vi "svc_Check for Waveform Parameter Continuity (no state).vi"(0 "scaled signal [EU]":waveform(dbl), 2 "checks for channel parameter change":T4, 5 "error in (no error)":errorcluster, 6 "reset":bool, 7 "expected channel info":T1={"sensor sensitivity"=1000.0, "engineering units"=1, "dB reference"=1.0, "custom label"="EU", "weighting filter"=0, "pregain"=0.0} {"pregain" format="%.2f"; "weighting filter" items=["Linear", "A-weighting", "B-weighting", "C-weighting", "ITU-R 468-4", "Dolby", "CCITT", "C-message", "Wb", "Wc", "Wd", "We", "Wf", "Wh", "Wj", "Wk", "Wm", "AES17 20 kHz lowpass", "AES17 40 kHz lowpass", "AES17 20 kHz highpass", "AES17 40 kHz highpass"]; "dB reference" format="%^.1e"; "engineering units" items=["custom..."=0, "V"=1, "A"=21, "C"=30, "pC"=31, "s"=32, "-"=29, "Pa"=2, "N"=20, "g"=3, "m/s^2"=4, "m/s"=5, "m"=6, "mm/s"=12, "mm"=13, "micron/s"=14, "micron"=15, "in/s^2"=7, "in/s"=8, "in"=9, "mil/s"=10, "mil"=11, "rad/s^2"=16, "rad/s"=17, "rad"=18, "deg/s^2"=26, "deg/s"=27, "deg"=28, "RPM"=22, "cycle/s^2"=23, "Hz"=24, "cycle"=25, "strain"=19]; "sensor sensitivity" format="%#_5f"}, 8 "channel index":i32, 9 "expected waveform parameters":T5) -> (11 "next expected waveform parameters":T5, 13 "next expected channel info":T1={"sensor sensitivity"=1000.0, "engineering units"=1, "dB reference"=1.0, "custom label"="EU", "weighting filter"=0, "pregain"=0.0} {"pregain" format="%.2f"; "weighting filter" items=["Linear", "A-weighting", "B-weighting", "C-weighting", "ITU-R 468-4", "Dolby", "CCITT", "C-message", "Wb", "Wc", "Wd", "We", "Wf", "Wh", "Wj", "Wk", "Wm", "AES17 20 kHz lowpass", "AES17 40 kHz lowpass", "AES17 20 kHz highpass", "AES17 40 kHz highpass"]; "dB reference" format="%^.1e"; "engineering units" items=["custom..."=0, "V"=1, "A"=21, "C"=30, "pC"=31, "s"=32, "-"=29, "Pa"=2, "N"=20, "g"=3, "m/s^2"=4, "m/s"=5, "m"=6, "mm/s"=12, "mm"=13, "micron/s"=14, "micron"=15, "in/s^2"=7, "in/s"=8, "in"=9, "mil/s"=10, "mil"=11, "rad/s^2"=16, "rad/s"=17, "rad"=18, "deg/s^2"=26, "deg/s"=27, "deg"=28, "RPM"=22, "cycle/s^2"=23, "Hz"=24, "cycle"=25, "strain"=19]; "sensor sensitivity" format="%#_5f"}, 14 "dup scaled signal [EU]":waveform(dbl), 15 "waveform parameter changed":bool, 16 "dt":dbl, 17 "array length":i32, 19 "error out":errorcluster)   [LabVIEW 2017]
uses:
  <vilib>/addons/_NISVFA/_Shared subVIs/Controls/svc_Waveform Parameters.ctl
  <vilib>/addons/_NISVFA/_Shared subVIs/Controls/svc_Channel Info.ctl
  <vilib>/addons/_NISVFA/_Shared subVIs/Controls/svc_Engineering Units Text Ring.ctl
  <vilib>/addons/_NISVFA/_Shared subVIs/Controls/svc_Weighting Filter Text Ring.ctl
  <vilib>/addons/_NISVFA/_Shared subVIs/Common/svc_Engineering Units to Unit Label.vi
  <vilib>/addons/_NISVFA/_Shared subVIs/Common/svc_Unit Label to Engineering Units.vi
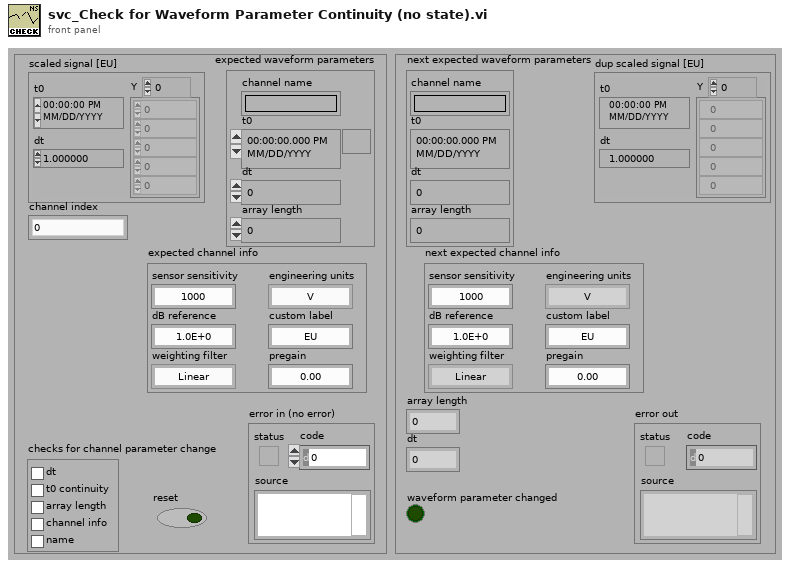
[diagram p1: front panel]
types:
  T1 = typedef "svc_Channel Info.ctl" = cluster{"sensor sensitivity":dbl, "engineering units":T2, "dB reference":dbl, "custom label":string, "weighting filter":T3, "pregain":dbl}
  T2 = typedef "svc_Engineering Units Text Ring.ctl" = u16
  T3 = typedef "svc_Weighting Filter Text Ring.ctl" = u16
  T4 = cluster{"dt":bool, "t0 continuity":bool, "array length":bool, "channel info":bool, "name":bool}
  T5 = typedef "svc_Waveform Parameters.ctl" = cluster{"channel name":string, "t0":timestamp, "dt":dbl, "array length":i32}
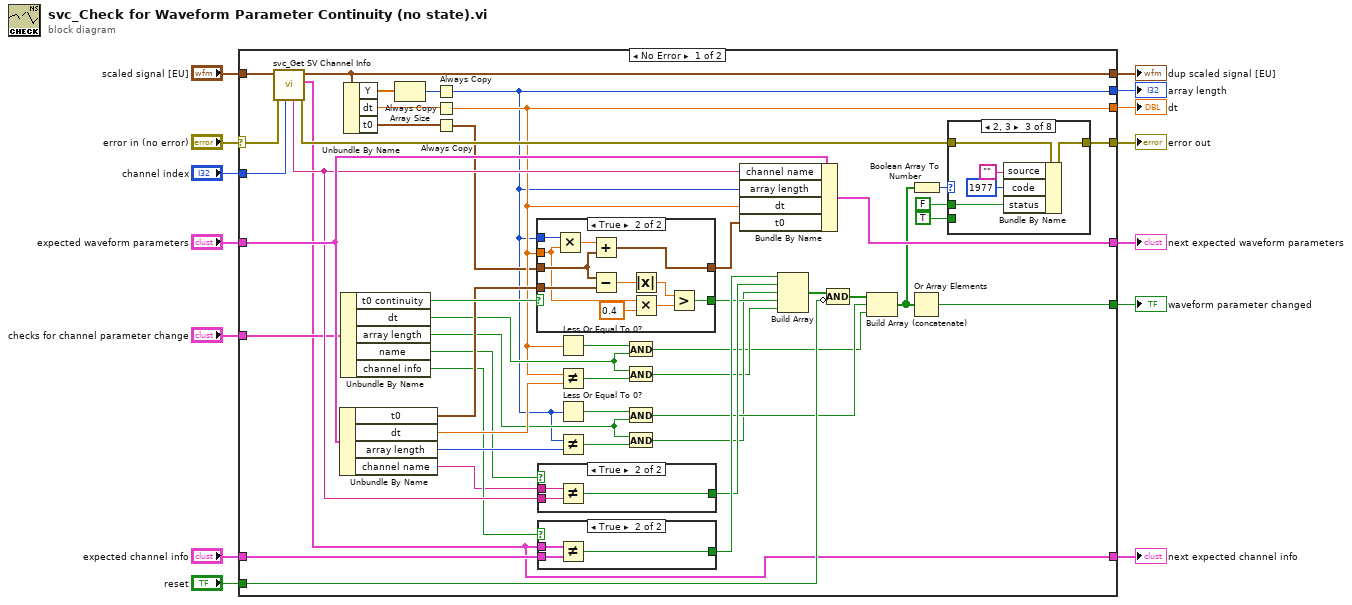
[diagram p0: block diagram]
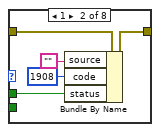
[diagram p3: hidden frame]
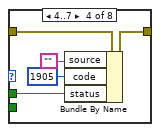
[diagram p4: hidden frame]
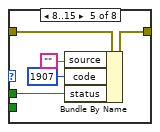
[diagram p5: hidden frame]
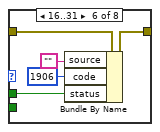
[diagram p6: hidden frame]
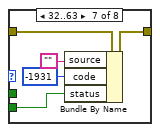
[diagram p7: hidden frame]
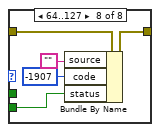
[diagram p8: hidden frame]
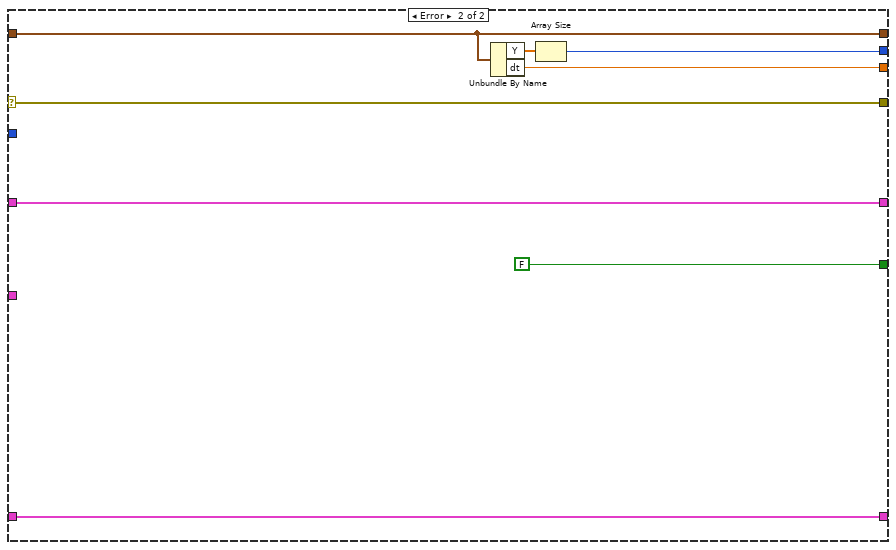
[diagram p12: hidden frame]
diagram:
  n1 = case shown="No Error" "error in (no error)" {
    selector: "error in (no error)" -> [w20 w121]
    tunnel: [w62 w121] -> w14
    tunnel: "expected waveform parameters" -> [w61 w127]
    tunnel: [w60 w127] -> w12
    tunnel: [w59 FALSE] -> w11
    tunnel: "reset" -> [w58 _]
    tunnel: "expected channel info" -> [w57 w126]
    tunnel: [w26 w126] -> w8
    tunnel: [w24 w125] -> w7
    tunnel: [w17 w122] -> w6
    tunnel: [w15 w123] -> w5
    tunnel: "channel index" -> [w54 _]
    tunnel: "checks for channel parameter change" -> [w53 _]
    tunnel: "scaled signal [EU]" -> [w52 w125]
    frame No Error {
      n2 = call <vilib>:"svc_Get SV Channel Info.vi"("channel index"=w54, "error in (no error)"=w20, "scaled signal [EU]"=w52) -> ("error out"=w56:errorcluster, "channel info"=w26:T1, "dup scaled signal [EU]"=w24:waveform(dbl), "channel name"=w55:string)  [unwired: 3 in, 2 out]
      n3 = Unbundle By Name(w61) -> ("t0"=w48:timestamp, "dt"=w49:dbl, "array length"=w51:i32, "channel name"=w44:string)
      n4 = Unbundle By Name(w53) -> ("t0 continuity"=w50:bool, "dt"=w19:bool, "array length"=w18:bool, "name"=w45:bool, "channel info"=w47:bool)
      n5 = Unbundle By Name ("Get Waveform Components")(w24) -> ("Y"=w25:dbl[], "dt"=w22:dbl, "t0"=w23:timestamp)
      n6 = Array Size(array=w25) -> (size(s)=w21:i32)
      n7 = Always Copy(1:w21) -> (0:w15:i32)
      n8 = Always Copy(1:w22) -> (0:w17:dbl)
      n9 = Always Copy(1:w23) -> (0:w16:timestamp)
      n10 = case shown="True" w50 {
        selector: w50 -> [w107 _]
        tunnel: [w107 w119] -> w38
        tunnel: w48 -> [_ w115]
        tunnel: w16 -> [w108 w114]
        tunnel: w15 -> [_ w113]
        tunnel: w17 -> [_ w112]
        tunnel: [w108 w109] -> w46
        frame False {
        }
        frame True {
          n11 = Multiply(x=w113, y=w112) -> (x*y=w118:dbl)
          n12 = Add(x=w118, y=w114) -> (x+y=w109:timestamp)
          n13 = Subtract(x=w114, y=w115) -> (x-y=w110:dbl)
          n14 = Absolute Value(x=w110) -> (abs(x)=w111:dbl)
          n15 = Multiply(x=w112, y=0.4 ("x")) -> (x*y=w116:dbl)
          n16 = Greater?(x=w111, y=w116) -> (0:w119:bool)
        }
      }
      n17 = case shown="True" w45 {
        selector: w45 -> [w99 _]
        tunnel: [w99 w102] -> w39
        tunnel: w55 -> [_ w101]
        tunnel: w44 -> [_ w100]
        frame False {
        }
        frame True {
          n18 = Not Equal?(x=w100, y=w101) -> (x != y?=w102:bool)
        }
      }
      n19 = case shown="True" w47 {
        selector: w47 -> [w103 _]
        tunnel: [w103 w106] -> w40
        tunnel: w57 -> [_ w105]
        tunnel: w26 -> [_ w104]
        frame False {
        }
        frame True {
          n20 = Not Equal?(x=w104, y=w105) -> (x != y?=w106:bool)
        }
      }
      n21 = Less Or Equal To 0?(x=w17) -> (x <= 0?=w28:bool)
      n22 = Not Equal?(x=w17, y=w49) -> (x != y?=w30:bool)
      n23 = Less Or Equal To 0?(x=w15) -> (x <= 0?=w34:bool)
      n24 = Not Equal?(x=w15, y=w51) -> (x != y?=w32:bool)
      n25 = And(x=w28, y=w19) -> (x .and. y?=w27:bool)
      n26 = And(x=w19, y=w30) -> (x .and. y?=w29:bool)
      n27 = And(x=w34, y=w18) -> (x .and. y?=w33:bool)
      n28 = And(x=w18, y=w32) -> (x .and. y?=w31:bool)
      n29 = Bundle By Name(cluster=w61, "channel name"=w55, "array length"=w15, "dt"=w17, "t0"=w46) -> (w60:T5)
      n30 = Build Array(w40, w39, w31, w38, w29) -> (w42:bool[])
      n31 = Compound Arithmetic op=AND(w42, invert w58) -> (w41:bool[])
      n32 = Build Array (concatenate)(w41, w33, w27) -> (w43:bool[])
      n33 = Or Array Elements(Boolean array=w43) -> (logical OR=w59:bool)
      n34 = Boolean Array To Number(Boolean array=w43) -> (number=w35:u32)
      n35 = case shown="2, 3" w35 {
        tunnel: w56 -> [w63 w68 w73 w78 w83 w88 w93 w98]
        tunnel: [w63 w67 w72 w77 w82 w87 w92 w97] -> w62
        tunnel: FALSE ("status") -> [_ w64 w69 w74 w79 w84 _ _]
        tunnel: TRUE ("status") -> [_ _ _ _ _ _ w90 w94]
        frame 0, Default {
        }
        frame 1 {
          n36 = Bundle By Name(cluster=w68, "source"="", "code"=1908, "status"=w64) -> (w67:errorcluster)
        }
        frame 2, 3 {
          n37 = Bundle By Name(cluster=w73, "source"="", "code"=1977, "status"=w69) -> (w72:errorcluster)
        }
        frame 4..7 {
          n38 = Bundle By Name(cluster=w78, "source"="", "code"=1905, "status"=w74) -> (w77:errorcluster)
        }
        frame 8..15 {
          n39 = Bundle By Name(cluster=w83, "source"="", "code"=1907, "status"=w79) -> (w82:errorcluster)
        }
        frame 16..31 {
          n40 = Bundle By Name(cluster=w88, "source"="", "code"=1906, "status"=w84) -> (w87:errorcluster)
        }
        frame 32..63 {
          n41 = Bundle By Name(cluster=w93, "source"="", "code"=-1931, "status"=w90) -> (w92:errorcluster)
        }
        frame 64..127 {
          n42 = Bundle By Name(cluster=w98, "source"="", "code"=-1907, "status"=w94) -> (w97:errorcluster)
        }
      }
    }
    frame Error {
      n43 = Unbundle By Name ("Get Waveform Components")(w125) -> ("Y"=w124:dbl[], "dt"=w122:dbl)
      n44 = Array Size(array=w124) -> (size(s)=w123:i32)
    }
  }
  "error out" <- w14
  "next expected waveform parameters" <- w12
  "waveform parameter changed" <- w11
  "next expected channel info" <- w8
  "dup scaled signal [EU]" <- w7
  "array length" <- w5
  "dt" <- w6
